vi "VisionRangingPose.vi"(5 "Turret Delta Y":dbl, 7 "Turret Delta X":dbl, 8 "Previous X Position (in)":dbl, 9 "Distance to Target (in)":dbl, 10 "Heading to Target (deg)":dbl, 11 "Previous Y Position (in)":dbl) -> (1 "Delta Y (in)":dbl, 2 "Delta X (in)":dbl)   [LabVIEW 2019]
doc: "Calculates the delta robot pose using the robot heading and the LimeLight ranging data."
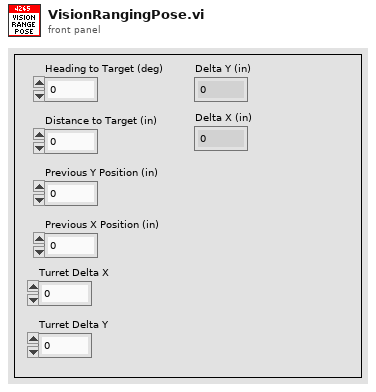
[diagram p1: front panel]
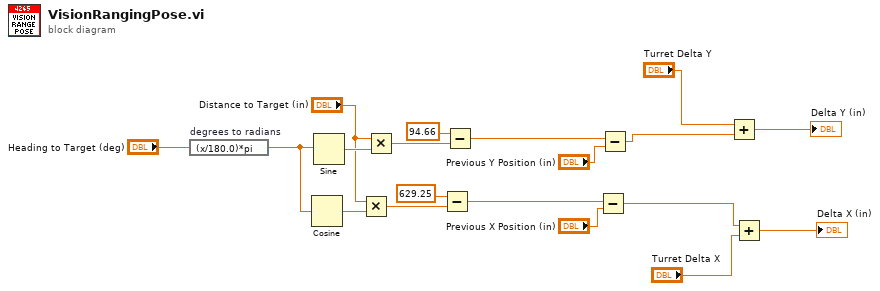
[diagram p0: block diagram]
diagram:
  n1 = expression code="(x/180.0)*pi" "degrees to radians"("Heading to Target (deg)") -> (w18:dbl)
  n2 = Cosine(x=w18) -> (cos(x)=w16:dbl)
  n3 = Sine(x=w18) -> (sin(x)=w17:dbl)
  n4 = Multiply(x="Distance to Target (in)", y=w16) -> (x*y=w11:dbl)
  n5 = Multiply(x="Distance to Target (in)", y=w17) -> (x*y=w13:dbl)
  n6 = Subtract(x=629.25, y=w11) -> (x-y=w8:dbl)
  n7 = Subtract(x=94.66, y=w13) -> (x-y=w10:dbl)
  n8 = Subtract(x=w8, y="Previous X Position (in)") -> (x-y=w3:dbl)
  n9 = Subtract(x=w10, y="Previous Y Position (in)") -> (x-y=w6:dbl)
  n10 = Add(x="Turret Delta Y", y=w6) -> (x+y=→"Delta Y (in)":dbl)
  n11 = Add(x=w3, y="Turret Delta X") -> (x+y=→"Delta X (in)":dbl)
